vi "HomeWork4.vi"() -> ()   [LabVIEW 2018]
uses:
  <vilib>/Analysis/NI_AALBase.lvlib
panel:
  out "Waveform Charging + Discharging":cluster{dbl, dbl}[](graph)
  out "Waveform Discharging":dbl[](graph)
  out "Waveform Charging":dbl[](graph)
  out "output waveform 2":waveform(dbl)
  out "output waveform":waveform(dbl)
  in  "amplitude 2":dbl=1.0 format="%0.2f"
  in  "amplitude":dbl=1.0 format="%0.2f"
  in  "stop":bool
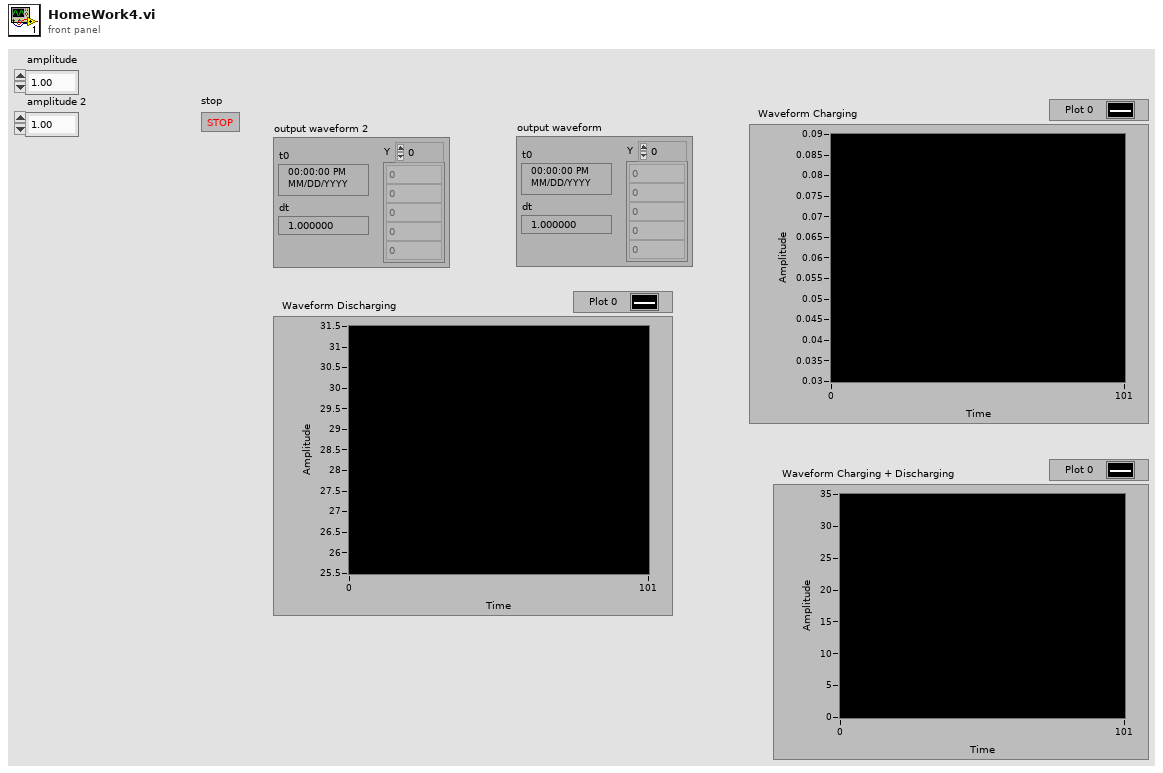
[diagram p1: front panel]
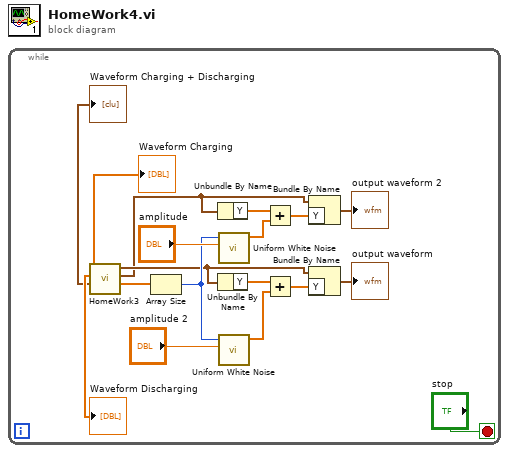
[diagram p0: block diagram]
diagram:
  n1 = while {
    stop <- "stop" stop-if-true
    n2 = call "HomeWork3.vi"() -> ("Waveform Charging"=→"Waveform Charging":dbl[], "Waveform Discharging"=→"Waveform Discharging":dbl[], "Waveform Charging + Discharging"=→"Waveform Charging + Discharging":cluster{dbl, dbl}[], "Discharging waveform"=w7:waveform(dbl), "Charging waveform"=w6:waveform(dbl), "Time array"=w16:dbl[])  [unwired: 5 in]
    n3 = Array Size(array=w16) -> (size(s)=w13:i32)
    n4 = Unbundle By Name(w6) -> ("Y"=w14:dbl[])
    n5 = Unbundle By Name(w7) -> ("Y"=w10:dbl[])
    n6 = call <vilib>:"Uniform White Noise.vi"("amplitude"="amplitude", "samples"=w13) -> ("uniform white noise"=w15:dbl[])  [unwired: 8 in, 1 out]
    n7 = call <vilib>:"Uniform White Noise.vi"("amplitude"="amplitude 2", "samples"=w13) -> ("uniform white noise"=w11:dbl[])  [unwired: 8 in, 1 out]
    n8 = Add(x=w14, y=w15) -> (x+y=w8:dbl[])
    n9 = Add(x=w10, y=w11) -> (x+y=w9:dbl[])
    n10 = Bundle By Name(cluster=w6, "Y"=w8) -> (→"output waveform 2":waveform(dbl))
    n11 = Bundle By Name(cluster=w7, "Y"=w9) -> (→"output waveform":waveform(dbl))
  }
